vi "Extract Sector and Image From Binary.vi"(0 "Binary Data(u64)":u64[](array[numeric]), 1 "Start Index":u64, 5 "# of u64 per image":u64, 7 "Height":i32, 9 "Width":i32, 11 "error in (no error)":errorcluster, 12 "Image Destination":T1) -> (4 "Image Out":T1, 6 "Left Sector":u16, 8 "Right Sector":u16, 15 "error out":errorcluster)   [LabVIEW 2013]
uses:
  <vilib>/vision/Image Controls.llb/IMAQ Image.ctl
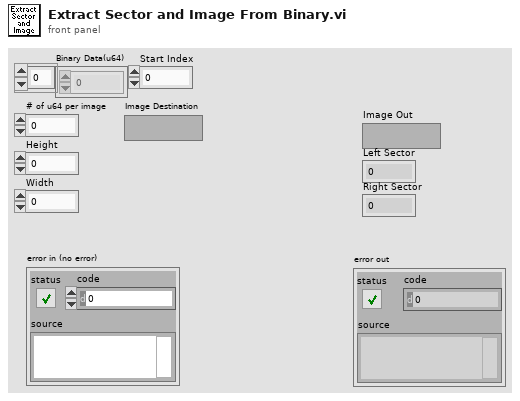
[diagram p1: front panel]
types:
  T1 = typedef "IMAQ Image.ctl" = refnum<image>
  T2 = enum16{"big-endian, network order", "native, host order", "little-endian"}
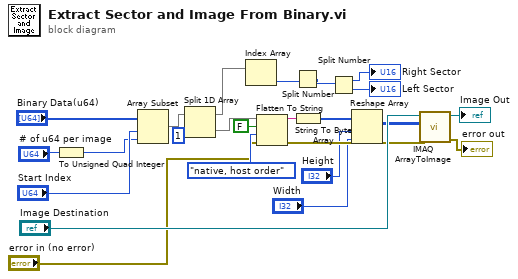
[diagram p0: block diagram]
diagram:
  n1 = To Unsigned Quad Integer(1:"# of u64 per image") -> (0:w16:u64)
  n2 = Array Subset(array="Binary Data(u64)", index="Start Index", length=w16) -> (w15:u64[])
  n3 = Split 1D Array(array=w15, index=1) -> (first subarray=w5:u64[], second subarray=w13:u64[])
  n4 = Index Array(array=w5) -> (element=w4:u64)  [unwired: 1 in]
  n5 = Flatten To String(anything=w13, prepend array or string size? (T)=FALSE, byte order (0:big-endian, network order)=T2."native, host order", error in (no error)="error in (no error)") -> (data string=w21:string, error out=w19:errorcluster)  [unwired: 1 out]
  n6 = Split Number(x=w4) -> (lo(x)=w3:u32)  [unwired: 1 out]
  n7 = String To Byte Array(string=w21) -> (unsigned byte array=w20:u8[])
  n8 = Split Number(x=w3) -> (hi(x)=→"Right Sector":u16, lo(x)=→"Left Sector":u16)
  n9 = Reshape Array(w20, "Height", "Width") -> (w18:u8[][])
  n10 = call "IMAQ ArrayToImage"("error in (no error)"=w19, "Image Pixels (U8)"=w18, "Image"="Image Destination") -> ("error out"=→"error out":errorcluster, "Image Out"=→"Image Out":T1)  [unwired: 7 in]
